vi "initialize.vi"(0 "HGF_SVVisitor_deregister":refnum<class "HGF_SVMonitorVisitor_deregister.lvclass">, 3 "initializationData":variant, 5 "error in (no error)":errorcluster, 7 "binaryString":string, 8 "I8 Array":i8[](array[numeric]), 9 "prependSize? (T)":bool, 11 "byteOrder (0:big-endian, network order)":T1(ring)) -> (14 "dup HGF_SVVisitor_deregister":refnum<class "HGF_SVMonitorVisitor_deregister.lvclass">, 17 "found?":bool, 19 "error out":errorcluster)   [LabVIEW 2012, in "HGF_SV.lvlib" / "HGF_SVMonitorVisitor_deregister.lvclass"]
doc: "This is a dynamic dispatch VI to be implemented by child classes to initialize their attributes.\n\n<B>Recommendation:</B> Use Variant for initialization data."
uses:
  HGF_SVMonitorVisitor_deregister.lvclass
  HGF_BaseClasses/HGF_NetworkVisitor/HGF_NetworkVisitor.lvclass
  HGF_BaseClasses/HGF_TriggeredEvent/HGF_TriggeredEvent.lvclass
  HGF_SVMonitorVisitor/HGF_SVMonitorVisitor.lvclass
  HGF_SVMonitorVisitor_deregister.lvclass/HGF_SVMonitorVisitor_deregister.ctl
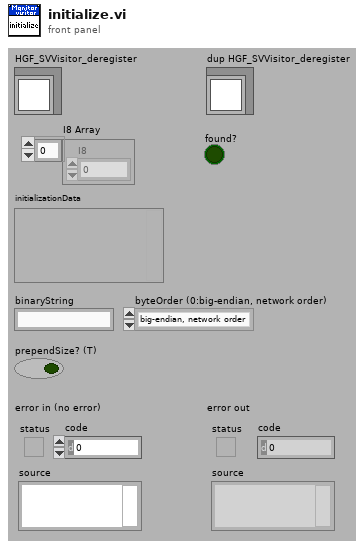
[diagram p1: front panel]
types:
  T1 = enum16{"big-endian, network order", "native, host order", "little-endian"}
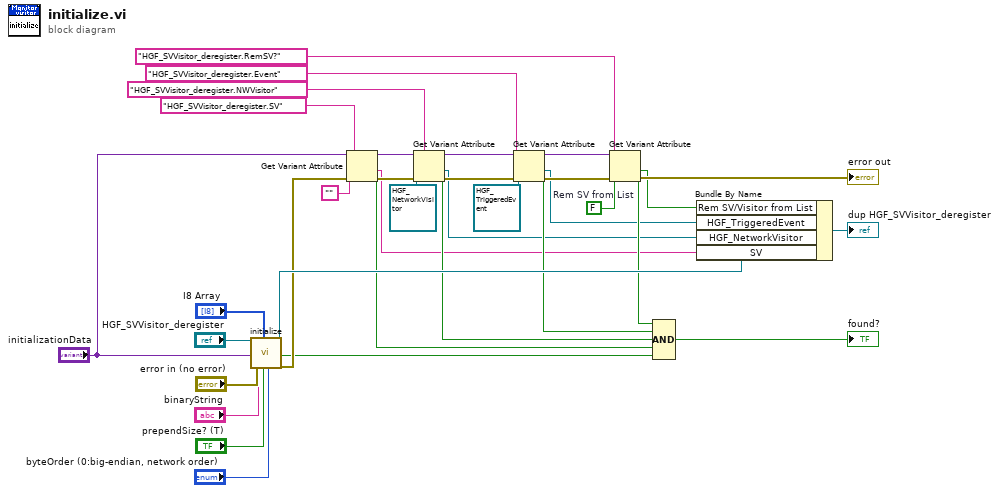
[diagram p0: block diagram]
diagram:
  w28 = FALSE  # Rem SV from List
  n1 = call-parent "initialize.vi"("HGF_Visitor"="HGF_SVVisitor_deregister", "initializationData"="initializationData", "error in (no error)"="error in (no error)", "binaryString"="binaryString", "I8 Array"="I8 Array", "prependSize? (T)"="prependSize? (T)", "byteOrder (0:big-endian, network order)"="byteOrder (0:big-endian, network order)") -> ("dup HGF_Visitor"=w29:refnum<class "HGF_SVMonitorVisitor_deregister.lvclass">, "found?"=w12:bool, "error out"=w14:errorcluster)  [unwired: 10 in]
  n2 = Get Variant Attribute(Variant="initializationData", name="HGF_SVVisitor_deregister.SV", default value (empty Variant)="", error in=w14) -> (duplicate Variant=w26:variant, found=w11:bool, value=w6:string, error out=w17:errorcluster)
  n3 = Get Variant Attribute(Variant=w26, name="HGF_SVVisitor_deregister.NWVisitor", default value (empty Variant)=refnum<class "HGF_NetworkVisitor.lvclass"> refnum ("HGF_NetworkVisitor"), error in=w17) -> (duplicate Variant=w25:variant, found=w10:bool, value=w5:refnum<class "HGF_NetworkVisitor.lvclass">, error out=w18:errorcluster)
  n4 = Get Variant Attribute(Variant=w25, name="HGF_SVVisitor_deregister.Event", default value (empty Variant)=refnum<class "HGF_TriggeredEvent.lvclass"> refnum ("HGF_BaseClasses.lvlib:HGF_TriggeredEvent.lvclass"), error in=w18) -> (duplicate Variant=w24:variant, found=w9:bool, value=w4:refnum<class "HGF_TriggeredEvent.lvclass">, error out=w19:errorcluster)
  n5 = Get Variant Attribute(Variant=w24, name="HGF_SVVisitor_deregister.RemSV?", default value (empty Variant)=w28, error in=w19) -> (found=w8:bool, value=w3:bool, error out=→"error out":errorcluster)  [unwired: 1 out]
  n6 = Compound Arithmetic op=AND(w8, w9, w10, w11, w12) -> (→"found?":bool)
  n7 = Bundle By Name(cluster=w29, "Rem SV/Visitor from List"=w3, "HGF_TriggeredEvent"=w4, "HGF_NetworkVisitor"=w5, "SV"=w6) -> (→"dup HGF_SVVisitor_deregister":refnum<class "HGF_SVMonitorVisitor_deregister.lvclass">)
